vi "Aiming.vi"(6 "PID Cluster":T2={"L1 to L4 PID Cluster"={"L1 PID Gains"={"Kp"=0.005, "Kd"=0.5, "Ki"=0.0005}, "L2 PID Gains"={"Kp"=0.01, "Kd"=1.0, "Ki"=0.005}, "L3 PID Gains"={"Kp"=0.05, "Kd"=1.0, "Ki"=0.0005}, "L4 PID Gains"={"Kp"=0.1, "Kd"=0.1, "Ki"=0.0005}}, "Stage PID Cluster"={"Stage Z PID"={"Kp"=0.0005, "Kd"=0.001, "Ki"=0.0}, "Stage Y PID"={"Kp"=0.0003, "Kd"=0.01, "Ki"=0.0}, "Stage X PID"={"Kp"=0.0003, "Kd"=0.01, "Ki"=0.0}}, "OCT Z PID Gains"={"Kp"=0.0003, "Kd"=0.0001, "Ki"=0.01}}, 7 "Offset Home 2 RCM":dbl[](array[numeric])=[0.0, 0.0, 0.0, 0.0], 8 "error in":errorcluster, 9 "Aiming Pt":dbl[](array[numeric])=[0.0, 0.0, 0.0, 0.0], 10 "Prev Posit Cluster":T3={"Prev L1 to L4 Posit"=[0.0, 0.0, 0.0, 0.0], "Prev Stage Posit"=[6.0, 6.0, 6.0], "Prev OCT Z Posit"=0.0}, 11 "FPGA VI Reference In":refnum<k20>) -> (0 "error out":errorcluster, 2 "Last Posit Cluster":T1={"Last L1 to L4 Posit"=[0.0, 0.0, 0.0, 0.0], "Last Stage Posit"=[6.0, 6.0, 6.0], "Last OCT Z Posit"=0.0}, 3 "FPGA VI Reference Out":refnum<k20>)   [LabVIEW 2016]
uses:
  <vilib>/Platform/TimedLoop/XDataNode/timing_clust.ctl
  <vilib>/Platform/TimedLoop/XDataNode/nitl_modes.ctl
  <vilib>/Platform/TimedLoop/XDataNode/wakeup.ctl
  Global Variables.vi
  <vilib>/platform/TimedLoop/XDataNode/XDataNode.xnode
  <vilib>/Platform/TimedLoop/XDataNode/XDNodeRunTimeDep.lvlib
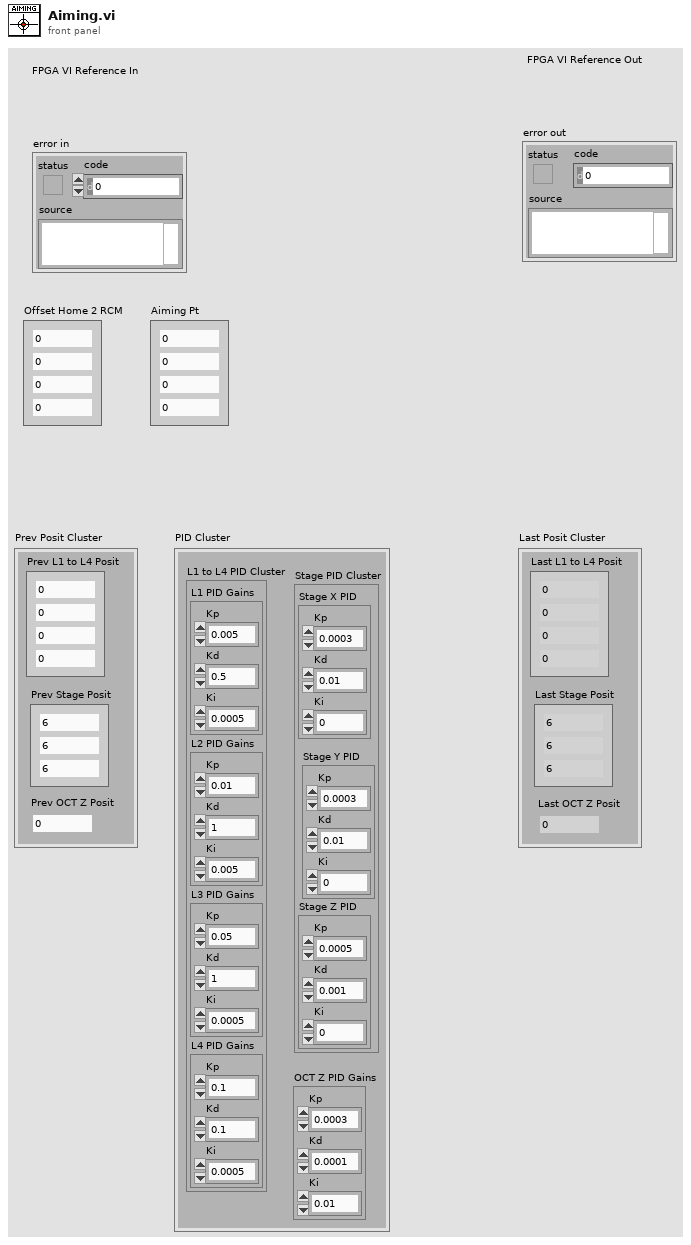
[diagram p1: front panel]
types:
  T1 = cluster{"Last L1 to L4 Posit":dbl[], "Last Stage Posit":dbl[], "Last OCT Z Posit":dbl}
  T2 = cluster{"L1 to L4 PID Cluster":cluster{"L1 PID Gains":cluster{"Kp":dbl, "Kd":dbl, "Ki":dbl}, "L2 PID Gains":cluster{"Kp":dbl, "Kd":dbl, "Ki":dbl}, "L3 PID Gains":cluster{"Kp":dbl, "Kd":dbl, "Ki":dbl}, "L4 PID Gains":cluster{"Kp":dbl, "Kd":dbl, "Ki":dbl}}, "Stage PID Cluster":cluster{"Stage Z PID":cluster{"Kp":dbl, "Kd":dbl, "Ki":dbl}, "Stage Y PID":cluster{"Kp":dbl, "Kd":dbl, "Ki":dbl}, "Stage X PID":cluster{"Kp":dbl, "Kd":dbl, "Ki":dbl}}, "OCT Z PID Gains":cluster{"Kp":dbl, "Kd":dbl, "Ki":dbl}}
  T3 = cluster{"Prev L1 to L4 Posit":dbl[], "Prev Stage Posit":dbl[], "Prev OCT Z Posit":dbl}
  T4 = cluster{"Stop Vacuum":bool, "Vacuum Force":i8, "Max Limit [mmHg]":dbl, "Slide in":i8, "Irrigation?":bool}
  T5 = typedef "XDNodeRunTimeDep.lvlib/timing_clust.ctl" = cluster{"Expected End [f-1]":u64, "Actual End [f-1]":u64, "Finished Late? [f-1]":bool, "Expected End [i-1]":u64, "Actual End [i-1]":u64, "Finished Late? [i-1]":bool, "Expected Start [i]":u64, "Actual Start [i]":u64, "Expected Start [f]":u64, "Actual Start [f]":u64, "Source Name":string, "Structure Name":string, "Period":i64, "Deadline":i64, "Offset":i64, "Start":i64, "Priority":i32, "Timeout":i32, "Mode":T6, "Wakeup Reason":T7, "Error":errorcluster, "Source Type":string, "Secondary Source Type":string, "Global End Time":u64, "Global Start Time":u64, "Frame Duration":u64, "Iteration Duration":u64, "Assigned CPU":i32, "I/O Scan Engine Mode":u32}
  T6 = typedef "XDNodeRunTimeDep.lvlib/nitl_modes.ctl" = enum32{"No Change", "Process missed periods, maintain original phase", "Discard missed periods, maintain original phase", "Process missed periods, ignore original phase", "Discard missed periods, ignore original phase"}
  T7 = typedef "XDNodeRunTimeDep.lvlib/wakeup.ctl" = enum32{"Normal", "Aborted", "Asynchronous wakeup", "Timing source error", "Timed loop error", "Timeout"}
  T8 = cluster{"Stage Z PID":cluster{"Kp":dbl, "Kd":dbl, "Ki":dbl}, "Stage Y PID":cluster{"Kp":dbl, "Kd":dbl, "Ki":dbl}, "Stage X PID":cluster{"Kp":dbl, "Kd":dbl, "Ki":dbl}}
  T9 = cluster{"L1 PID Gains":cluster{"Kp":dbl, "Kd":dbl, "Ki":dbl}, "L2 PID Gains":cluster{"Kp":dbl, "Kd":dbl, "Ki":dbl}, "L3 PID Gains":cluster{"Kp":dbl, "Kd":dbl, "Ki":dbl}, "L4 PID Gains":cluster{"Kp":dbl, "Kd":dbl, "Ki":dbl}}
  T10 = cluster{"Accurus button":bool[], "Accurus engaged?":bool, "Vacuum Force":i32, "Accurus Ch. A Vout":dbl, "Accurus Ch. B Vout":dbl, "Irrigation engaged?":bool}
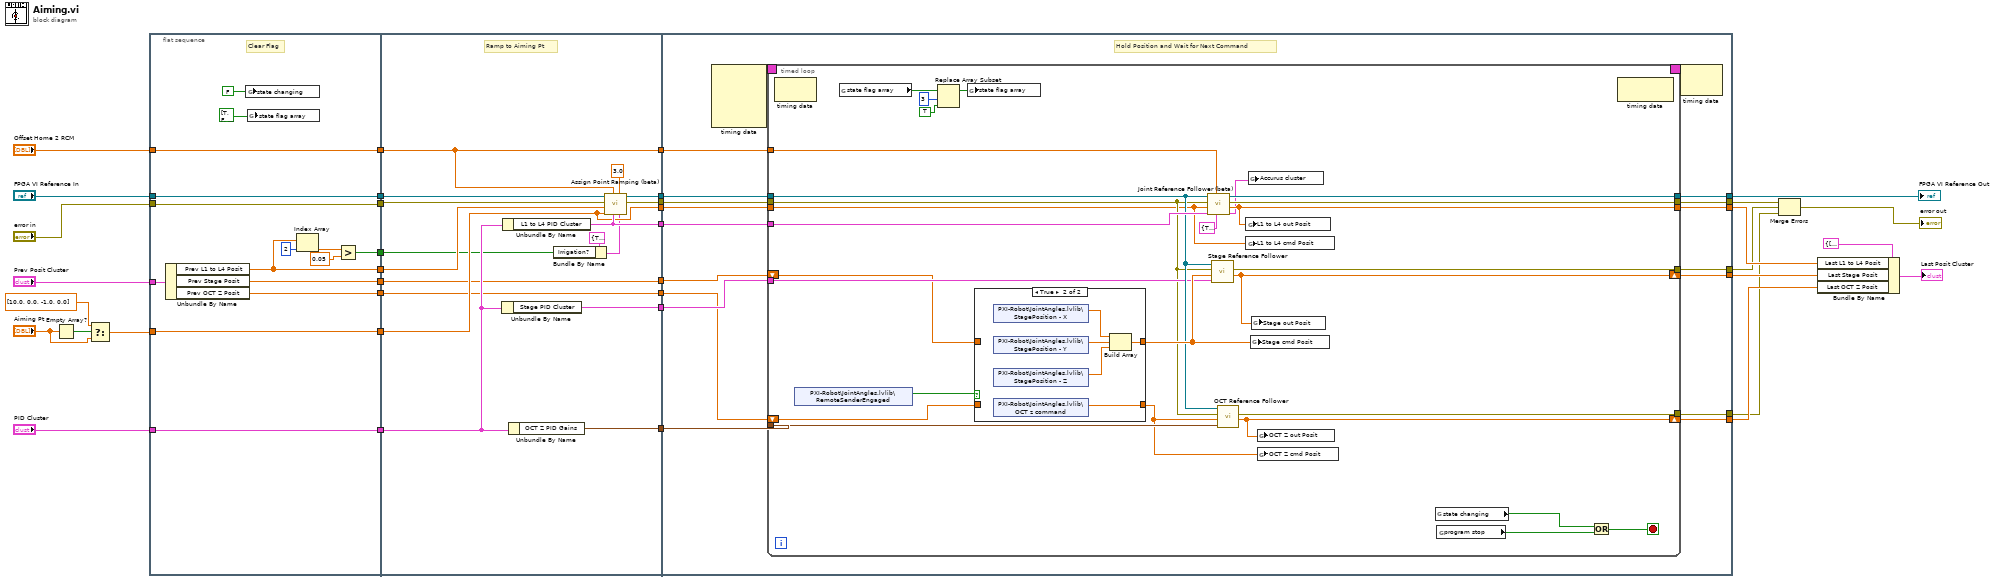
[diagram p0: block diagram]
diagram:
  n1 = Empty Array?(array="Aiming Pt") -> (empty?=w29:bool)
  n2 = Select(t=dbl[] [10.0, 0.0, -1.0, 0.0] ("First Trk Pt 2"), s=w29, f="Aiming Pt") -> (s? t:f=w26:dbl[])
  n3 = flat-sequence {
    tunnel: [w50] -> w37
    tunnel: "FPGA VI Reference In" -> [w50]
    tunnel: "error in" -> [w49]
    tunnel: [w49] -> w36
    tunnel: [w42] -> w35
    tunnel: "PID Cluster" -> [w47]
    tunnel: "Offset Home 2 RCM" -> [w48]
    tunnel: [w48] -> w33
    tunnel: [w43] -> w31
    tunnel: w26 -> [w43]
    tunnel: [w47] -> w19
    tunnel: "Prev Posit Cluster" -> [w46]
    tunnel: [w45] -> w5
    tunnel: [w44] -> w2
    tunnel: [w38] -> w1
    tunnel: w37 -> [w69]
    tunnel: w36 -> [w68]
    tunnel: w35 -> [w66]
    tunnel: w33 -> [w63]
    tunnel: w31 -> [w58]
    tunnel: [w65] -> w30
    tunnel: [w58] -> w25
    tunnel: [w64] -> w24
    tunnel: [w63] -> w23
    tunnel: [w62] -> w22
    tunnel: w19 -> [w60]
    tunnel: [w61] -> w18
    tunnel: [w59] -> w17
    tunnel: w5 -> [w57]
    tunnel: [w57] -> w4
    tunnel: [w56] -> w3
    tunnel: w2 -> [w56]
    tunnel: w1 -> [w53]
    tunnel: [w81] -> w13
    tunnel: [w80] -> w8
    tunnel: w30 -> [w84]
    tunnel: w25 -> [w83]
    tunnel: w24 -> [w85]
    tunnel: w23 -> [w72]
    tunnel: w22 -> [w82]
    tunnel: [w79] -> w20
    tunnel: [w78] -> w21
    tunnel: w18 -> [w77]
    tunnel: w17 -> [w76]
    tunnel: [w75] -> w14
    tunnel: [w74] -> w7
    tunnel: [w73] -> w6
    tunnel: w4 -> [w71]
    tunnel: w3 -> [w70]
    frame #0 {
      # "Clear Flag"
      n4 = Unbundle By Name(w46) -> ("Prev L1 to L4 Posit"=w42:dbl[], "Prev Stage Posit"=w45:dbl[], "Prev OCT Z Posit"=w44:dbl)
      n5 = global write "Global Variables.vi" "state changing"(FALSE ("state changing")) -> ()
      n6 = global write "Global Variables.vi" "state flag array"(bool[] [TRUE, FALSE, FALSE, FALSE, FALSE, FALSE, FALSE, FALSE, FALSE] ("state flag array")) -> ()
      n7 = Index Array(array=w42, index=2) -> (element=w40:dbl)
      n8 = Greater?(x=w40, y=0.05) -> (0:w38:bool)
    }
    frame #1 {
      # "Ramp to Aiming Pt"
      n9 = Unbundle By Name(w60) -> ("Stage PID Cluster"=w61:T8)
      n10 = Unbundle By Name(w60) -> ("L1 to L4 PID Cluster"=w62:T9)
      n11 = Unbundle By Name(w60) -> ("OCT Z PID Gains"=w59:cluster{"Kp":dbl, "Kd":dbl, "Ki":dbl})
      n12 = Bundle By Name(cluster=T4 {"Stop Vacuum"=TRUE, "Vacuum Force"=0, "Max Limit [mmHg]"=600.0, "Slide in"=0, "Irrigation?"=FALSE} ("Accurus Ctrl Cluster"), "Irrigation?"=w53) -> (w54:T4)
      n13 = call "Assign Point Ramping (beta).vi"("Accurus Ctrl Cluster"=w54, "Ramp Time [sec]"=3.0, "L1 to L4 PID Cluster"=w62, "Offset Home2RCM"=w63, "Destination Posit Array [mm]"=w58, "Previous Posit Array"=w66, "error in"=w68, "FPGA VI Reference In"=w69) -> ("error out"=w65:errorcluster, "FPGA VI Reference Out"=w64:refnum<k20>)  [unwired: 1 in, 1 out]
    }
    frame #2 {
      # "Hold Position and Wait for Next Command"
      n14 = node-c288() -> (w87:T5)  [unwired: 4 in]
      n15 = timed-loop {
        timing: w87 -> [_]
        timing-out: [_] -> w86
        tunnel: w85 -> [w104]
        tunnel: w84 -> [w96]
        tunnel: w72 -> [w110]
        tunnel: w83 -> [w90]
        tunnel: w82 -> [w109]
        tunnel: [w108] -> w81
        tunnel: [w107] -> w80
        tunnel: [w102] -> w79
        tunnel: w77 -> [w101]
        tunnel: w76 -> [w100]
        tunnel: [w95] -> w74
        tunnel: [w94] -> w73
        shift-right: [w105] -> w78
        shift-left: w71 -> [w92]
        shift-right: [w99] -> w75
        shift-left: w70 -> [w91]
        stop <- w97 stop-if-true
        n16 = node-c288() -> ()  [unwired: 1 in, 1 out]
        n17 = shared-variable "PXI-Robot\\JointAngles.lvlib\\RemoteSenderEngaged"() -> (w93:bool)  [unwired: 1 in, 1 out]
        n18 = global read "Global Variables.vi" "state flag array"() -> (w114:bool[])
        n19 = Replace Array Subset(array=w114, new element=TRUE ("new element/subarray"), index=3) -> (w113:bool[])
        n20 = global write "Global Variables.vi" "state flag array"(w113) -> ()
        n21 = case shown="True" w93 {
          tunnel: [w117 w119] -> w106
          tunnel: [w116 w118] -> w98
          tunnel: w92 -> [w117 _]
          tunnel: w91 -> [w116 _]
          frame False {
            # "Hold Position if not Engaged"
          }
          frame True {
            n22 = shared-variable "PXI-Robot\\JointAngles.lvlib\\StagePosition - X"() -> (w122:dbl)  [unwired: 1 in, 1 out]
            n23 = shared-variable "PXI-Robot\\JointAngles.lvlib\\StagePosition - Y"() -> (w121:dbl)  [unwired: 1 in, 1 out]
            n24 = shared-variable "PXI-Robot\\JointAngles.lvlib\\StagePosition - Z"() -> (w120:dbl)  [unwired: 1 in, 1 out]
            n25 = shared-variable "PXI-Robot\\JointAngles.lvlib\\OCT z command"() -> (w118:dbl)  [unwired: 1 in, 1 out]
            n26 = Build Array(w122, w121, w120) -> (w119:dbl[])
          }
        }
        n27 = call "Joint Reference Follower (beta).vi"("Accurus Ctrl Cluster"=T4 {"Stop Vacuum"=TRUE, "Vacuum Force"=0, "Max Limit [mmHg]"=600.0, "Slide in"=0, "Irrigation?"=FALSE}, "Offset Home2RCM [deg/mm]"=w110, "PID Ctrl Cluster"=w109, "Ref Array [deg/mm]"=w90, "error in"=w96, "FPGA VI Reference In"=w104) -> ("Accurus Output Cluster"=w88:T10, "Output Posit Array [deg/mm]"=w102:dbl[], "error out"=w107:errorcluster, "FPGA VI Reference Out"=w108:refnum<k20>)  [unwired: 2 in]
        n28 = call "Stage Reference Follower.vi"("Stage PID Cluster"=w101, "Stage cmd Posit [mm]"=w106, "error in"=w96, "FPGA VI Reference In"=w104) -> ("Stage out Posit [mm]"=w105:dbl[], "error out"=w95:errorcluster)  [unwired: 5 in, 1 out]
        n29 = call "OCT Reference Follower.vi"("OCT Z PID Gains"=w100, "OCT  Z cmd Posit [mm]"=w98, "error in"=w96, "FPGA VI Reference In"=w104) -> ("OCT  Z out Posit [mm]"=w99:dbl, "error out"=w94:errorcluster)  [unwired: 5 in, 1 out]
        n30 = global write "Global Variables.vi" "L1 to L4 out Posit"(w102) -> ()
        n31 = global write "Global Variables.vi" "L1 to L4 cmd Posit"(w90) -> ()
        n32 = global write "Global Variables.vi" "Accurus cluster"(w88) -> ()
        n33 = global write "Global Variables.vi" "Stage cmd Posit"(w106) -> ()
        n34 = global write "Global Variables.vi" "Stage out Posit"(w105) -> ()
        n35 = global write "Global Variables.vi" "OCT Z out Posit"(w99) -> ()
        n36 = global write "Global Variables.vi" "OCT Z cmd Posit"(w98) -> ()
        n37 = global read "Global Variables.vi" "state changing"() -> (w115:bool)
        n38 = global read "Global Variables.vi" "program stop"() -> (w103:bool)
        n39 = Or(x=w115, y=w103) -> (x .or. y?=w97:bool)
        n40 = node-c288() -> ()  [unwired: 1 in, 1 out]
      }
      n41 = node-c288(w86) -> ()  [unwired: 1 out]
    }
  }
  n42 = Merge Errors(w8, w7, w6) -> (→"error out":errorcluster)
  n43 = Bundle By Name(cluster=T1 {"Last L1 to L4 Posit"=[0.0, 0.0, 0.0, 0.0], "Last Stage Posit"=[6.0, 6.0, 6.0], "Last OCT Z Posit"=0.0} ("Last Posit Cluster 2"), "Last L1 to L4 Posit"=w20, "Last Stage Posit"=w21, "Last OCT Z Posit"=w14) -> (→"Last Posit Cluster":T1)
  "FPGA VI Reference Out" <- w13
